vi "Test_TCP Handshake.vi"() -> ()   [LabVIEW 2013]
uses:
  Connection/auth -- cluster.ctl
  <vilib>/LabVIEW Open Source Project/Unicity/RandomStringGenerator/RandomStringGenerator.lvclass
  Connection/Connection.lvclass
  <vilib>/LabVIEW Open Source Project/OpenURI/openURI.lvlib
panel:
  out "State verfied":bool
  out "Echo":string
  out "Echo verfied":bool
  out "Auth Ack/Nack":string
  out "Challenge verified":bool
  out "error out 2":errorcluster
  out "error out":errorcluster
  out "Client Reader":string
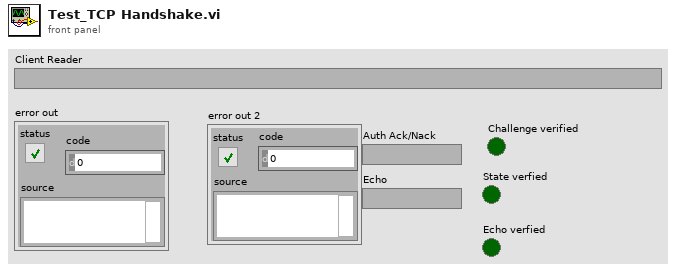
[diagram p1: front panel]
types:
  T1 = enum16{"Standard", "Buffered", "CRLF", "Immediate"}
  T2 = typedef "Connection_GOSPL.lvlib/Connection.lvclass/auth -- cluster.ctl" = cluster{"URL":string, "username":string, "state":string}
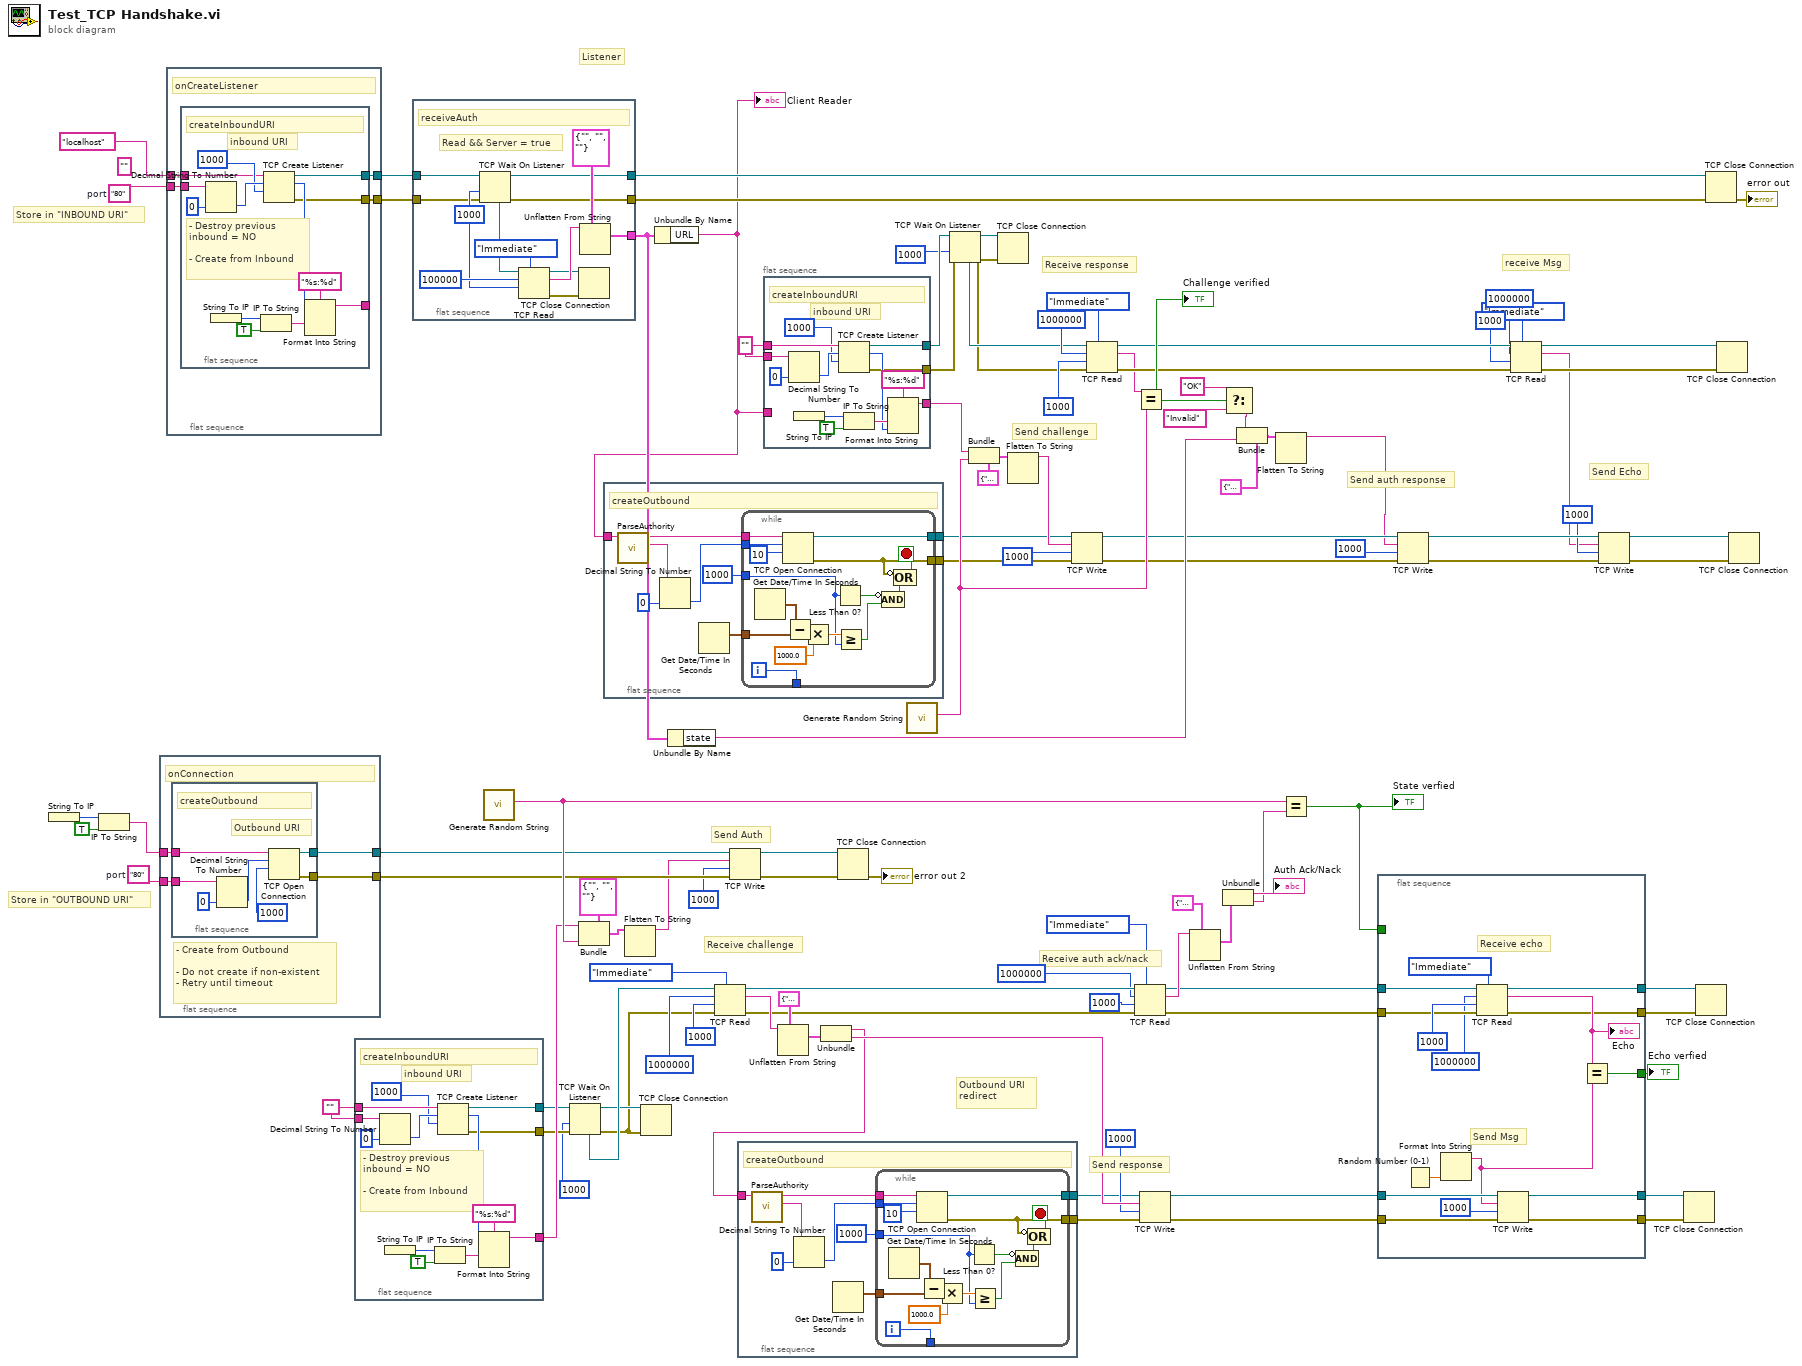
[diagram p0: block diagram]
diagram:
  (unwired) ""
  w36 = ""
  w38 = ""
  w80 = "80"  # port
  w85 = "80"  # port
  # "receive Msg"
  # "Store in \"OUTBOUND URI\""
  # "Store in \"INBOUND URI\""
  # "Listener"
  # "Outbound URI\nredirect"
  # "Send Echo"
  # "Receive auth ack/nack"
  # "Send auth response"
  # "Receive response"
  # "Send response"
  # "Receive challenge"
  # "Send challenge"
  # "Send Auth"
  n1 = String To IP() -> (0:w4:u32)  [unwired: 1 in]
  n2 = IP To String(1:TRUE ("dot notation? (F)"), 2:w4) -> (0:w1:string)
  n3 = flat-sequence {
    tunnel: [w109] -> w79
    tunnel: [w108] -> w78
    tunnel: w80 -> [w107]
    tunnel: w1 -> [w106]
    frame #0 {
      # "- Create from Outbound\n\n- Do not create if non-existent\n- Retry until timeout"
      # "onConnection"
      n4 = flat-sequence {
        tunnel: [w114] -> w109
        tunnel: [w113] -> w108
        tunnel: w107 -> [w112]
        tunnel: w106 -> [w110]
        frame #0 {
          # "Outbound URI"
          # "createOutbound"
          n5 = Decimal String To Number(string=w112, default (0L)=u16 0 ("port")) -> (number=w115:u16)  [unwired: 1 in, 1 out]
          n6 = TCP Open Connection(address=w110, remote port or service name=w115, timeout ms (60000)=1000 ("timeout in ms (-1)")) -> (connection ID=w114:refnum<k5>, error out=w113:errorcluster)  [unwired: 2 in]
        }
      }
    }
  }
  n7 = flat-sequence {
    tunnel: w85 -> [w120]
    tunnel: [w119] -> w84
    tunnel: [w118] -> w30
    tunnel: "localhost" ("name") -> [w117]
    frame #0 {
      # "onCreateListener"
      n8 = flat-sequence {
        tunnel: w120 -> [w133]
        tunnel: [w130] -> w119
        tunnel: [w123] -> _
        tunnel: [w122] -> w118
        tunnel: w117 -> [w121]
        frame #0 {
          # "- Destroy previous\ninbound = NO\n\n- Create from Inbound"
          # "inbound URI"
          # "createInboundURI"
          n9 = Decimal String To Number(string=w133, default (0L)=u16 0 ("port")) -> (number=w132:u16)  [unwired: 1 in, 1 out]
          n10 = String To IP() -> (0:w128:u32)  [unwired: 1 in]
          n11 = IP To String(1:TRUE ("dot notation? (F)"), 2:w128) -> (0:w126:string)
          n12 = TCP Create Listener(9:1000 ("timeout in ms (-1)"), 10:w132, 11:w121) -> (0:w122:errorcluster, 2:w124:u16, 3:w130:refnum<k5>)  [unwired: 2 in]
          n13 = Format Into String(format string="%s:%d", w126, w124) -> (resulting string=w123:string)  [unwired: 2 in, 1 out]
        }
      }
    }
  }
  n14 = flat-sequence {
    tunnel: w38 -> [w146]
    tunnel: w38 -> [w145]
    tunnel: [w142] -> w16
    tunnel: [w135] -> w37
    tunnel: [w134] -> w15
    frame #0 {
      # "- Destroy previous\ninbound = NO\n\n- Create from Inbound"
      # "inbound URI"
      # "createInboundURI"
      n15 = Decimal String To Number(string=w145, default (0L)=u16 0 ("port")) -> (number=w144:u16)  [unwired: 1 in, 1 out]
      n16 = String To IP() -> (0:w140:u32)  [unwired: 1 in]
      n17 = IP To String(1:TRUE ("dot notation? (F)"), 2:w140) -> (0:w138:string)
      n18 = TCP Create Listener(9:1000 ("timeout in ms (-1)"), 10:w144, 11:w146) -> (0:w134:errorcluster, 2:w136:u16, 3:w142:refnum<k5>)  [unwired: 2 in]
      n19 = Format Into String(format string="%s:%d", w138, w136) -> (resulting string=w135:string)  [unwired: 2 in, 1 out]
    }
  }
  n20 = flat-sequence {
    tunnel: [w159] -> w87
    tunnel: [w156] -> w83
    tunnel: [w151] -> w82
    tunnel: w84 -> [w157]
    tunnel: w30 -> [w147]
    frame #0 {
      w152 = 1000 ("timeout in ms (-1)")
      # "Read && Server = true"
      # "receiveAuth"
      n21 = TCP Wait On Listener(8:w147, 9:w152, 11:w157) -> (0:w151:errorcluster, 3:w156:refnum<k5>, 4:w155:refnum<k5>)  [unwired: 1 in, 2 out]
      n22 = TCP Read(connection ID=w155, bytes to read=100000 ("timeout in ms (-1)"), 7:T1."Immediate" ("mode (standard)"), 9:w152) -> (connection ID out=w148:refnum<k5>, data out=w150:string, error out=w149:errorcluster)  [unwired: 1 in]
      n23 = TCP Close Connection(connection ID=w148, error in (no error)=w149) -> ()  [unwired: 1 in, 2 out]
      n24 = Unflatten From String(type=T2 {"URL"="", "username"="", "state"=""} ("Authorization"), binary string=w150) -> (value=w159:T2)  [unwired: 3 in, 2 out]
    }
  }
  n25 = call <vilib>:"Generate Random String.vi"() -> ("Random String"=w88:string)  [unwired: 11 in]
  n26 = TCP Wait On Listener(8:w15, 9:1000 ("timeout in ms (-1)"), 11:w16) -> (0:w13:errorcluster, 3:w14:refnum<k5>, 4:w17:refnum<k5>)  [unwired: 1 in, 2 out]
  n27 = Bundle(cluster=T2 {"URL"="", "username"="", "state"=""} ("Authorization"), "URL"=w37, "state"=w88) -> (w97:T2)  [unwired: 1 in]
  n28 = flat-sequence {
    tunnel: w27 -> [w162]
    tunnel: [w161] -> w29
    tunnel: [w160] -> w28
    frame #0 {
      # "createOutbound"
      n29 = call <vilib>:"ParseAuthority.vi"("authority"=w162) -> ("port"=w166:string, "host"=w163:string)  [unwired: 7 in, 2 out]
      n30 = Decimal String To Number(string=w166, default (0L)=u16 0 ("port")) -> (number=w164:u16)  [unwired: 1 in, 1 out]
      n31 = Get Date/Time In Seconds() -> (seconds since 1Jan1904=w168:timestamp)
      n32 = while {
        tunnel: [w173] -> w161
        tunnel: 1000 ("timeout in ms (-1)") -> [w176]
        tunnel: w168 -> [w184]
        tunnel: w164 -> [w175]
        tunnel: w163 -> [w171]
        tunnel: [w170] -> w160
        tunnel: [w169] -> _
        i -> [w169]
        stop <- w172 stop-if-true
        n33 = Get Date/Time In Seconds() -> (seconds since 1Jan1904=w183:timestamp)
        n34 = TCP Open Connection(address=w171, remote port or service name=w175, timeout ms (60000)=10 ("timeout in ms (-1)")) -> (connection ID=w173:refnum<k5>, error out=w170:errorcluster)  [unwired: 2 in]
        n35 = Subtract(x=w183, y=w184) -> (x-y=w182:dbl)
        n36 = Multiply(x=w182, y=1000.0) -> (x*y=w180:dbl)
        n37 = Less Than 0?(x=w176) -> (x < 0?=w177:bool)
        n38 = Greater Or Equal?(x=w180, y=w176) -> (x >= y?=w179:bool)
        n39 = Compound Arithmetic op=AND(invert w177, w179) -> (w178:bool)
        n40 = Compound Arithmetic op=OR(invert w170, w178) -> (w172:bool)
      }
    }
  }
  n41 = Flatten To String(anything=w97) -> (data string=w77:string)  [unwired: 3 in, 2 out]
  n42 = TCP Close Connection(connection ID=w14, error in (no error)=w13) -> ()  [unwired: 1 in, 2 out]
  n43 = Unbundle By Name(w87) -> ("URL"=w27:string)
  "Client Reader" <- w27
  n44 = Unbundle By Name(w87) -> ("state"=w86:string)
  n45 = TCP Read(connection ID=w17, bytes to read=1000000 ("timeout in ms (-1)"), error in (no error)=w13, 7:T1."Immediate" ("mode (standard)"), 9:1000 ("timeout in ms (-1)")) -> (connection ID out=w66:refnum<k5>, data out=w70:string, error out=w67:errorcluster)
  n46 = TCP Write(connection ID=w79, data in=w77, error in (no error)=w78, 9:1000 ("timeout in ms (-1)")) -> (connection ID out=w75:refnum<k5>, error out=w74:errorcluster)  [unwired: 1 out]
  n47 = flat-sequence {
    tunnel: w26 -> [w187]
    tunnel: [w186] -> w25
    tunnel: [w185] -> w24
    frame #0 {
      # "createOutbound"
      n48 = call <vilib>:"ParseAuthority.vi"("authority"=w187) -> ("port"=w191:string, "host"=w188:string)  [unwired: 7 in, 2 out]
      n49 = Decimal String To Number(string=w191, default (0L)=u16 0 ("port")) -> (number=w189:u16)  [unwired: 1 in, 1 out]
      n50 = Get Date/Time In Seconds() -> (seconds since 1Jan1904=w193:timestamp)
      n51 = while {
        tunnel: [w198] -> w186
        tunnel: 1000 ("timeout in ms (-1)") -> [w201]
        tunnel: w193 -> [w209]
        tunnel: w189 -> [w200]
        tunnel: w188 -> [w196]
        tunnel: [w195] -> w185
        tunnel: [w194] -> _
        i -> [w194]
        stop <- w197 stop-if-true
        n52 = Get Date/Time In Seconds() -> (seconds since 1Jan1904=w208:timestamp)
        n53 = TCP Open Connection(address=w196, remote port or service name=w200, timeout ms (60000)=10 ("timeout in ms (-1)")) -> (connection ID=w198:refnum<k5>, error out=w195:errorcluster)  [unwired: 2 in]
        n54 = Subtract(x=w208, y=w209) -> (x-y=w207:dbl)
        n55 = Multiply(x=w207, y=1000.0) -> (x*y=w205:dbl)
        n56 = Less Than 0?(x=w201) -> (x < 0?=w202:bool)
        n57 = Greater Or Equal?(x=w205, y=w201) -> (x >= y?=w204:bool)
        n58 = Compound Arithmetic op=AND(invert w202, w204) -> (w203:bool)
        n59 = Compound Arithmetic op=OR(invert w195, w203) -> (w197:bool)
      }
    }
  }
  n60 = flat-sequence {
    tunnel: w36 -> [w222]
    tunnel: w36 -> [w221]
    tunnel: [w218] -> w10
    tunnel: [w212] -> w35
    tunnel: [w211] -> w8
    tunnel: w27 -> [_]
    frame #0 {
      # "inbound URI"
      # "createInboundURI"
      n61 = Decimal String To Number(string=w221, default (0L)=u16 0 ("port")) -> (number=w220:u16)  [unwired: 1 in, 1 out]
      n62 = String To IP() -> (0:w217:u32)  [unwired: 1 in]
      n63 = TCP Create Listener(9:1000 ("timeout in ms (-1)"), 10:w220, 11:w222) -> (0:w211:errorcluster, 2:w213:u16, 3:w218:refnum<k5>)  [unwired: 2 in]
      n64 = IP To String(1:TRUE ("dot notation? (F)"), 2:w217) -> (0:w215:string)
      n65 = Format Into String(format string="%s:%d", w215, w213) -> (resulting string=w212:string)  [unwired: 2 in, 1 out]
    }
  }
  n66 = Unflatten From String(type=cluster{"redirect":string, "challenge":string} {"redirect"="", "challenge"=""} ("cluster"), binary string=w70) -> (value=w103:cluster{"redirect":string, "challenge":string})  [unwired: 3 in, 2 out]
  n67 = Unbundle(w103) -> ("redirect"=w26:string, "challenge"=w44:string)
  n68 = TCP Close Connection(connection ID=w75, error in (no error)=w74) -> (error out=→"error out 2":errorcluster)  [unwired: 1 in, 1 out]
  n69 = call <vilib>:"Generate Random String.vi"() -> ("Random String"=w60:string)  [unwired: 11 in]
  n70 = TCP Wait On Listener(8:w8, 9:1000 ("timeout in ms (-1)"), 11:w10) -> (0:w9:errorcluster, 3:w12:refnum<k5>, 4:w11:refnum<k5>)  [unwired: 1 in, 2 out]
  n71 = Bundle(cluster=cluster{"redirect":string, "challenge":string} {"redirect"="", "challenge"=""}, "redirect"=w35, "challenge"=w60) -> (w105:cluster{"redirect":string, "challenge":string})
  n72 = TCP Close Connection(connection ID=w12, error in (no error)=w9) -> ()  [unwired: 1 in, 2 out]
  n73 = Flatten To String(anything=w105) -> (data string=w58:string)  [unwired: 3 in, 2 out]
  n74 = TCP Write(connection ID=w29, data in=w58, error in (no error)=w28, 9:1000 ("timeout in ms (-1)")) -> (connection ID out=w57:refnum<k5>, error out=w51:errorcluster)  [unwired: 1 out]
  n75 = TCP Read(connection ID=w11, bytes to read=1000000 ("timeout in ms (-1)"), error in (no error)=w9, 7:T1."Immediate" ("mode (standard)"), 9:1000 ("timeout in ms (-1)")) -> (connection ID out=w42:refnum<k5>, data out=w34:string, error out=w39:errorcluster)
  n76 = TCP Read(connection ID=w66, bytes to read=1000000 ("timeout in ms (-1)"), error in (no error)=w67, 7:T1."Immediate" ("mode (standard)"), 9:1000 ("timeout in ms (-1)")) -> (connection ID out=w65:refnum<k5>, data out=w68:string, error out=w64:errorcluster)
  n77 = Equal?(x=w34, y=w60) -> (x = y?=w102:bool)
  "Challenge verified" <- w102
  n78 = TCP Write(connection ID=w25, data in=w44, error in (no error)=w24, 9:1000 ("timeout in ms (-1)")) -> (connection ID out=w48:refnum<k5>, error out=w45:errorcluster)  [unwired: 1 out]
  n79 = Unflatten From String(type=cluster{"response":string, "header":string} {"response"="", "header"=""} ("cluster"), binary string=w68) -> (value=w92:cluster{"response":string, "header":string})  [unwired: 3 in, 2 out]
  n80 = Unbundle(w92) -> ("response"=→"Auth Ack/Nack":string, "header"=w90:string)
  n81 = Select(t="OK", s=w102, f="Invalid") -> (s? t:f=w94:string)
  n82 = Bundle(cluster=cluster{"response":string, "header":string} {"response"="", "header"=""}, "response"=w94, "header"=w86) -> (w95:cluster{"response":string, "header":string})
  n83 = Flatten To String(anything=w95) -> (data string=w52:string)  [unwired: 3 in, 2 out]
  n84 = Equal?(x=w88, y=w90) -> (x = y?=w5:bool)
  "State verfied" <- w5
  n85 = flat-sequence {
    tunnel: [w238] -> w99
    tunnel: w65 -> [w235]
    tunnel: w64 -> [w234]
    tunnel: [w231] -> w62
    tunnel: [w230] -> w61
    tunnel: w48 -> [w229]
    tunnel: [w228] -> w47
    tunnel: [w227] -> w46
    tunnel: w45 -> [w226]
    tunnel: w5 -> [_]
    frame #0 {
      # "Send Msg"
      # "Receive echo"
      n86 = Random Number (0-1)() -> (number: 0 to 1=w237:dbl)
      n87 = Format Into String(w237) -> (resulting string=w225:string)  [unwired: 3 in, 1 out]
      n88 = TCP Read(connection ID=w235, bytes to read=1000000 ("timeout in ms (-1)"), error in (no error)=w234, 7:T1."Immediate" ("mode (standard)"), 9:1000 ("timeout in ms (-1)")) -> (connection ID out=w231:refnum<k5>, data out=w233:string, error out=w230:errorcluster)
      "Echo" <- w233
      n89 = TCP Write(connection ID=w229, data in=w225, error in (no error)=w226, 9:1000 ("timeout in ms (-1)")) -> (connection ID out=w228:refnum<k5>, error out=w227:errorcluster)  [unwired: 1 out]
      n90 = Equal?(x=w233, y=w225) -> (x = y?=w238:bool)
    }
  }
  n91 = TCP Write(connection ID=w57, data in=w52, error in (no error)=w51, 9:1000 ("timeout in ms (-1)")) -> (connection ID out=w56:refnum<k5>, error out=w50:errorcluster)  [unwired: 1 out]
  n92 = TCP Read(connection ID=w42, bytes to read=1000000 ("timeout in ms (-1)"), error in (no error)=w39, 7:T1."Immediate" ("mode (standard)"), 9:1000 ("timeout in ms (-1)")) -> (connection ID out=w41:refnum<k5>, data out=w32:string, error out=w40:errorcluster)
  n93 = TCP Write(connection ID=w56, data in=w32, error in (no error)=w50, 9:1000 ("timeout in ms (-1)")) -> (connection ID out=w55:refnum<k5>, error out=w49:errorcluster)  [unwired: 1 out]
  n94 = TCP Close Connection(connection ID=w47, error in (no error)=w46) -> ()  [unwired: 1 in, 2 out]
  n95 = TCP Close Connection(connection ID=w62, error in (no error)=w61) -> ()  [unwired: 1 in, 2 out]
  n96 = TCP Close Connection(connection ID=w83, error in (no error)=w82) -> (error out=→"error out":errorcluster)  [unwired: 1 in, 1 out]
  n97 = TCP Close Connection(connection ID=w41, error in (no error)=w40) -> ()  [unwired: 1 in, 2 out]
  n98 = TCP Close Connection(connection ID=w55, error in (no error)=w49) -> ()  [unwired: 1 in, 2 out]
  "Echo verfied" <- w99
